vi "PerfAddRemove.vi"() -> (3 "Add time":dbl format="%.2p")   [LabVIEW 2024, in "VarCircularBuffer.Tests.Perf.lvlib"]
uses:
  VarCircularBuffer.Tests.Perf.lvlib
  VarCircularBuffer.lvclass/VarCircularBuffer.ctl
  <vilib>/Analysis/baseanly.llb/Mean (DBL).vi
  IsFull.vi
  <vilib>/Analysis/NI_AALBase.lvlib
  VarCircularBuffer.lvclass
panel:
  out "remove time":dbl format="%.2p"
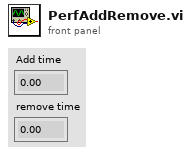
[diagram p1: front panel]
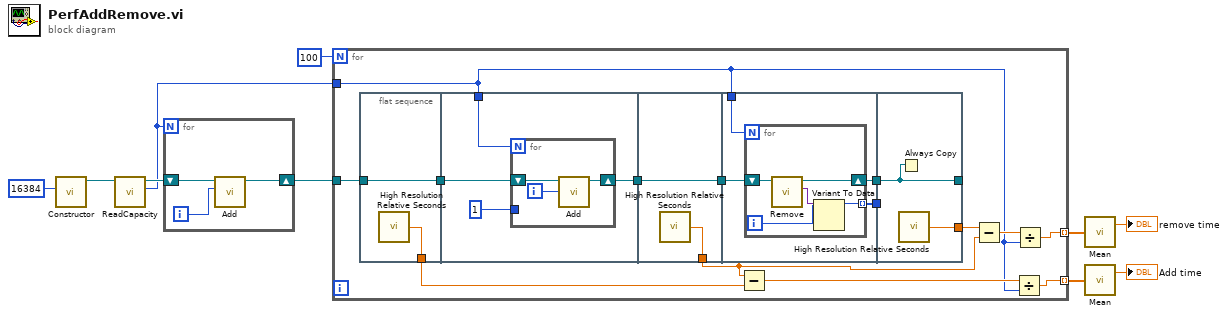
[diagram p0: block diagram]
diagram:
  n1 = call "Constructor.vi"("Capacity"=u32 16384) -> ("TypedCircularBuffer out"=w4:refnum<class "VarCircularBuffer.lvclass">)  [unwired: 10 in]
  n2 = call "ReadCapacity.vi"("TypedCircularBuffer in"=w4) -> ("capacity"=w1:u32, "TypedCircularBuffer out"=w3:refnum<class "VarCircularBuffer.lvclass">)  [unwired: 9 in]
  n3 = for {
    N: w1 -> [_]
    shift-right: [w11] -> w2
    shift-left: w3 -> [w13]
    i -> [w12]
    n4 = call "Add.vi"("Element"=w12, "TypedCircularBuffer in"=w13) -> ("TypedCircularBuffer out"=w11:refnum<class "VarCircularBuffer.lvclass">)  [unwired: 7 in, 2 out]
  }
  n5 = for {
    N: 100 -> [_]
    tunnel: [w17] -> w10 mode=indexing
    tunnel: w2 -> [w26]
    tunnel: [w18] -> w5 mode=indexing
    tunnel: w1 -> [w14]
    n6 = flat-sequence {
      tunnel: w26 -> [w29]
      tunnel: [w29] -> w23
      tunnel: [w28] -> w21
      tunnel: [w32] -> w24
      tunnel: w23 -> [w33]
      tunnel: w14 -> [w31]
      tunnel: [w38] -> w22
      tunnel: [w37] -> w25
      tunnel: w24 -> [w37]
      tunnel: w25 -> [w42]
      tunnel: w14 -> [w41]
      tunnel: [w40] -> w16
      tunnel: [w39] -> w15
      tunnel: [w49] -> w27
      tunnel: [w48] -> _
      tunnel: w16 -> [w48]
      tunnel: w15 -> [_]
      frame #0 {
        n7 = call <vilib>:"High Resolution Relative Seconds.vi"() -> ("relative seconds"=w28:dbl)
      }
      frame #1 {
        n8 = for {
          N: w31 -> [_]
          shift-right: [w35] -> w32
          shift-left: w33 -> [w36]
          tunnel: 1 -> [_]
          i -> [w34]
          n9 = call "Add.vi"("Element"=w34, "TypedCircularBuffer in"=w36) -> ("TypedCircularBuffer out"=w35:refnum<class "VarCircularBuffer.lvclass">)  [unwired: 7 in, 2 out]
        }
      }
      frame #2 {
        n10 = call <vilib>:"High Resolution Relative Seconds.vi"() -> ("relative seconds"=w38:dbl)
      }
      frame #3 {
        n11 = for {
          N: w41 -> [_]
          shift-right: [w46] -> w40
          shift-left: w42 -> [w47]
          tunnel: [w43] -> w39 mode=indexing
          i -> [w44]
          n12 = call "Remove.vi"("TypedCircularBuffer in"=w47) -> ("element"=w45:variant, "TypedCircularBuffer out"=w46:refnum<class "VarCircularBuffer.lvclass">)  [unwired: 8 in, 1 out]
          n13 = Variant To Data(type=w44, Variant=w45) -> (data=w43:i32)  [unwired: 1 in, 1 out]
        }
      }
      frame #4 {
        n14 = Always Copy(1:w48) -> ()  [unwired: 1 out]
        n15 = call <vilib>:"High Resolution Relative Seconds.vi"() -> ("relative seconds"=w49:dbl)
      }
    }
    n16 = Subtract(x=w22, y=w21) -> (x-y=w19:dbl)
    n17 = Subtract(x=w27, y=w22) -> (x-y=w20:dbl)
    n18 = Divide(x=w19, y=w14) -> (x/y=w18:dbl)
    n19 = Divide(x=w20, y=w14) -> (x/y=w17:dbl)
  }
  n20 = call-poly <vilib>:"Mean.vi"("X"=w10) -> ("mean"=→"remove time":dbl)  [unwired: 1 out]
  n21 = call-poly <vilib>:"Mean.vi"("X"=w5) -> ("mean"=→"Add time":dbl)  [unwired: 1 out]
